vi "home.vi"   [LabVIEW 2011]
types:
  T1 = typedef "WPI_DigitalInputDevRef.ctl" = cluster{"DevStatus":errorcluster, "DIO Channel":T2, "Digital Module":T3}
  T2 = typedef "FPGA_DIOChannel.ctl" = enum8{"DIO 1", "DIO 2", "DIO 3", "DIO 4", "DIO 5", "DIO 6", "DIO 7", "DIO 8", "DIO 9", "DIO 10", "DIO 11", "DIO 12", "DIO 13", "DIO 14", "Invalid"}
  T3 = typedef "FPGA_TypedefDigitalModule.ctl" = enum16{"Digital Module 1", "Digital Module 2"}
  T4 = typedef "WPI_MotorControlDeviceRef.ctl" = cluster{"DeviceStatus":errorcluster, "Type":enum16{"PWM", "CAN"}, "PWM":cluster{"Digital Module":T3, "PWM Channel":T5, "DeadBand":T6}, "CAN":cluster{"Device Number":u8, "Control Mode":T7, "Semaphore":T8, "Max Vout":dbl}, "Invert":bool, "TransformRef":T9, "InvTransformRef":T9}
  T5 = typedef "FPGA_DIOPWMChannel.ctl" = enum8{"PWM 1", "PWM 2", "PWM 3", "PWM 4", "PWM 5", "PWM 6", "PWM 7", "PWM 8", "PWM 9", "PWM 10", "Invalid"}
  T6 = typedef "WPI_PWMDeadband.ctl" = cluster{"Name":string, "maxPositivePwm":i32, "minPositivePwm":i32, "centerPwm":i32, "maxNegativePwm":i32, "minNegativePwm":i32, "angularRange":u16}
  T7 = typedef "WPI_CANJaguar_ControlMode.ctl" = enum8{"Percent VBus", "Current", "Speed", "Position", "Voltage"}
  T8 = typedef "Semaphore RefNum" = refnum<k1>
  T9 = typedef "WPI_PWMTransform_ConPane.ctl" = refnum<vi>
  T10 = typedef "WPI_EncoderDevRef.ctl" = cluster{"DevStatus":errorcluster, "EncoderIndex":T11, "CounterIndex":T12, "DistancePerCount":dbl, "Decoding Type":T13}
  T11 = typedef "FPGA_EncoderIdx.ctl" = enum8{"Enc 0", "Enc 1", "Enc 2", "Enc 3", "Invalid"}
  T12 = typedef "FPGA_CounterCtrSystemIndex.ctl" = enum8{"Ctr 0", "Ctr 1", "Ctr 2", "Ctr 3", "Ctr 4", "Ctr 5", "Ctr 6", "Ctr 7", "Invalid"}
  T13 = typedef "WPI_EncoderType.ctl" = enum16{"1x", "2x", "4x"}
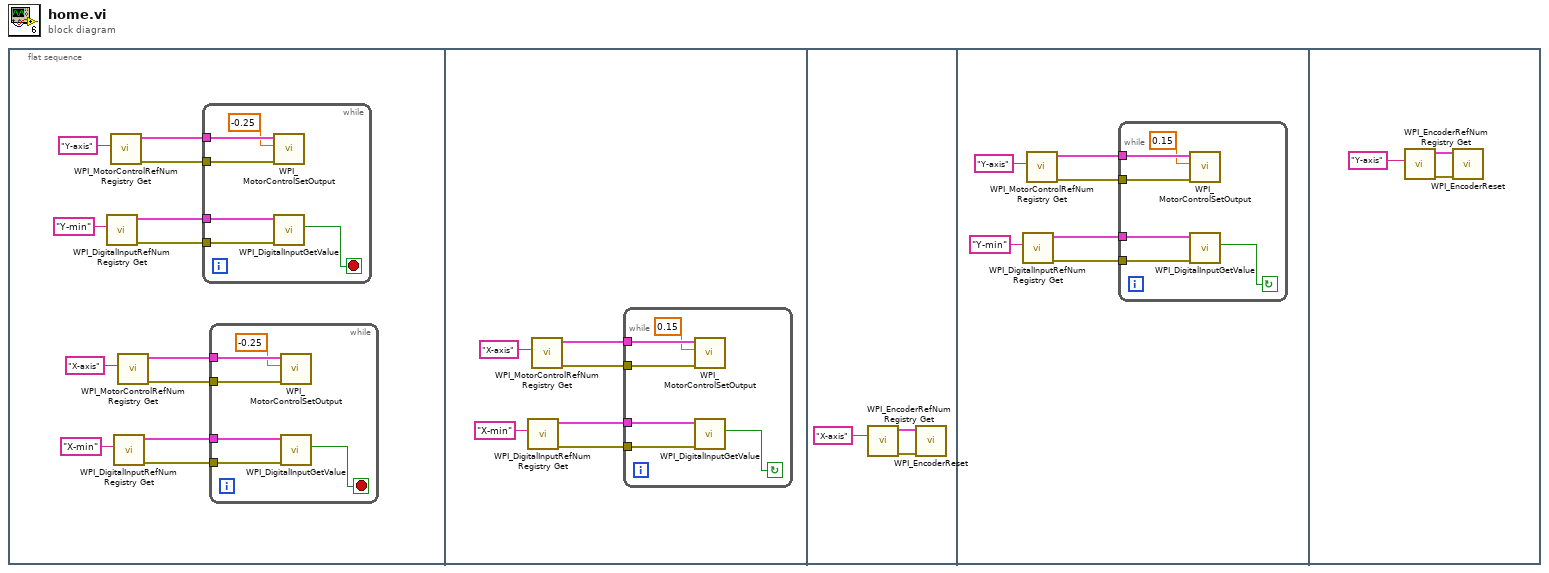
[diagram p0: block diagram]
diagram:
  n1 = flat-sequence {
    frame #0 {
      n2 = call <vilib>:"WPI_DigitalInputRefNum Registry Get.vi"("refnum name"="Y-min") -> ("error out"=w2:errorcluster, "DigitalInputDevRef"=w3:T1)  [unwired: 9 in]
      n3 = call <vilib>:"WPI_MotorControlRefNum Registry Get.vi"("refnum name"="Y-axis") -> ("error out"=w4:errorcluster, "MotorControlDevRef"=w5:T4)  [unwired: 9 in]
      n4 = call <vilib>:"WPI_DigitalInputRefNum Registry Get.vi"("refnum name"="X-min") -> ("error out"=w8:errorcluster, "DigitalInputDevRef"=w9:T1)  [unwired: 9 in]
      n5 = call <vilib>:"WPI_MotorControlRefNum Registry Get.vi"("refnum name"="X-axis") -> ("error out"=w10:errorcluster, "MotorControlDevRef"=w11:T4)  [unwired: 9 in]
      n6 = while {
        tunnel: w5 -> [w18]
        tunnel: w4 -> [w17]
        tunnel: w3 -> [w15]
        tunnel: w2 -> [w14]
        stop <- w13 stop-if-true
        n7 = call <vilib>:"WPI_MotorControlSetOutput.vi"("error in (no error)"=w17, "Output"=-0.25, "MotorControlDevRef"=w18) -> ()  [unwired: 7 in, 2 out]
        n8 = call <vilib>:"WPI_DigitalInputGetValue.vi"("error in (no error)"=w14, "DigitalInputDevRef"=w15) -> ("Value"=w13:bool)  [unwired: 7 in, 2 out]
      }
      n9 = while {
        tunnel: w11 -> [w24]
        tunnel: w10 -> [w23]
        tunnel: w9 -> [w21]
        tunnel: w8 -> [w20]
        stop <- w19 stop-if-true
        n10 = call <vilib>:"WPI_MotorControlSetOutput.vi"("error in (no error)"=w23, "Output"=-0.25, "MotorControlDevRef"=w24) -> ()  [unwired: 7 in, 2 out]
        n11 = call <vilib>:"WPI_DigitalInputGetValue.vi"("error in (no error)"=w20, "DigitalInputDevRef"=w21) -> ("Value"=w19:bool)  [unwired: 7 in, 2 out]
      }
    }
    frame #1 {
      n12 = call <vilib>:"WPI_DigitalInputRefNum Registry Get.vi"("refnum name"="X-min") -> ("error out"=w29:errorcluster, "DigitalInputDevRef"=w28:T1)  [unwired: 9 in]
      n13 = call <vilib>:"WPI_MotorControlRefNum Registry Get.vi"("refnum name"="X-axis") -> ("error out"=w27:errorcluster, "MotorControlDevRef"=w26:T4)  [unwired: 9 in]
      n14 = while {
        tunnel: w26 -> [w36]
        tunnel: w27 -> [w35]
        tunnel: w28 -> [w33]
        tunnel: w29 -> [w32]
        stop <- w31 continue-if-true
        n15 = call <vilib>:"WPI_MotorControlSetOutput.vi"("error in (no error)"=w35, "Output"=0.15, "MotorControlDevRef"=w36) -> ()  [unwired: 7 in, 2 out]
        n16 = call <vilib>:"WPI_DigitalInputGetValue.vi"("error in (no error)"=w32, "DigitalInputDevRef"=w33) -> ("Value"=w31:bool)  [unwired: 7 in, 2 out]
      }
    }
    frame #2 {
      n17 = call <vilib>:"WPI_EncoderRefNum Registry Get.vi"("refnum name"="X-axis") -> ("error out"=w38:errorcluster, "EncoderDevRef"=w39:T10)  [unwired: 9 in]
      n18 = call <vilib>:"WPI_EncoderReset.vi"("error in (no error)"=w38, "EncoderDevRef"=w39) -> ()  [unwired: 8 in, 2 out]
    }
    frame #3 {
      n19 = call <vilib>:"WPI_DigitalInputRefNum Registry Get.vi"("refnum name"="Y-min") -> ("error out"=w41:errorcluster, "DigitalInputDevRef"=w42:T1)  [unwired: 9 in]
      n20 = call <vilib>:"WPI_MotorControlRefNum Registry Get.vi"("refnum name"="Y-axis") -> ("error out"=w43:errorcluster, "MotorControlDevRef"=w44:T4)  [unwired: 9 in]
      n21 = while {
        tunnel: w44 -> [w51]
        tunnel: w43 -> [w50]
        tunnel: w42 -> [w48]
        tunnel: w41 -> [w47]
        stop <- w46 continue-if-true
        n22 = call <vilib>:"WPI_MotorControlSetOutput.vi"("error in (no error)"=w50, "Output"=0.15, "MotorControlDevRef"=w51) -> ()  [unwired: 7 in, 2 out]
        n23 = call <vilib>:"WPI_DigitalInputGetValue.vi"("error in (no error)"=w47, "DigitalInputDevRef"=w48) -> ("Value"=w46:bool)  [unwired: 7 in, 2 out]
      }
    }
    frame #4 {
      n24 = call <vilib>:"WPI_EncoderRefNum Registry Get.vi"("refnum name"="Y-axis") -> ("error out"=w53:errorcluster, "EncoderDevRef"=w52:T10)  [unwired: 9 in]
      n25 = call <vilib>:"WPI_EncoderReset.vi"("error in (no error)"=w53, "EncoderDevRef"=w52) -> ()  [unwired: 8 in, 2 out]
    }
  }
